vi "Set Picture.File Path.vi"(8 "error in (no error)":errorcluster, 10 "Picture.File Path":path, 11 "xwpfRun.Figure in":refnum<class "xwpfRun.Figure.lvclass">) -> (0 "error out":errorcluster, 3 "xwpfRun.Figure out":refnum<class "xwpfRun.Figure.lvclass">)   [LabVIEW 2017, in "Word_Specific.lvlib" / "xwpfRun.Figure.lvclass"]
uses:
  xwpfRun.Figure.lvclass
  xwpfRun.Figure.lvclass/xwpfRun.Figure.ctl
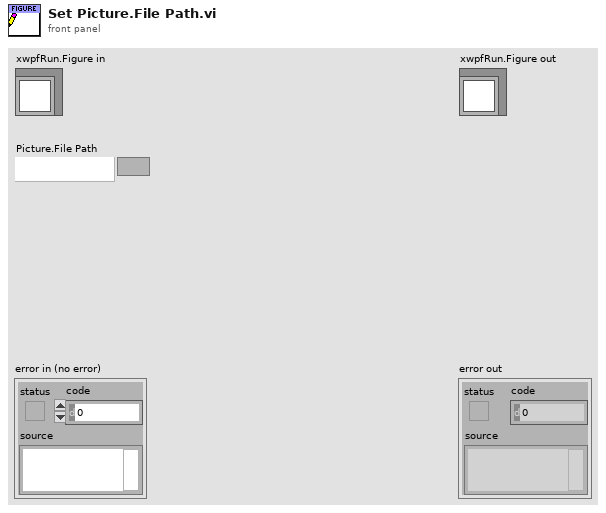
[diagram p1: front panel]
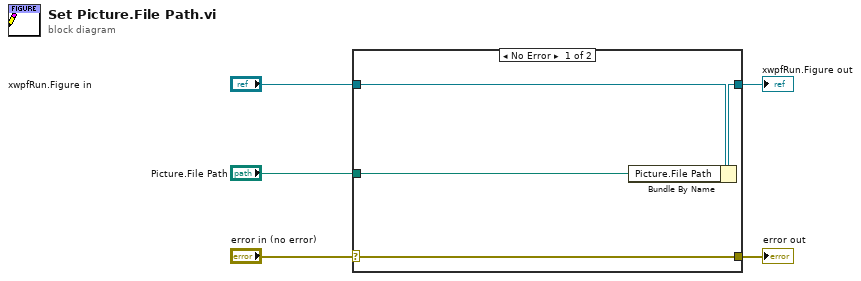
[diagram p0: block diagram]
diagram:
  n1 = case shown="No Error" "error in (no error)" {
    selector: "error in (no error)" -> [w9 w10]
    tunnel: [w9 w10] -> w4
    tunnel: [w7 w11] -> w2
    tunnel: "xwpfRun.Figure in" -> [w8 w11]
    tunnel: "Picture.File Path" -> [w6 _]
    frame No Error {
      n2 = Bundle By Name(cluster=w8, "Picture.File Path"=w6) -> (w7:refnum<class "xwpfRun.Figure.lvclass">)
    }
    frame Error {
    }
  }
  "error out" <- w4
  "xwpfRun.Figure out" <- w2
